vi "Configure Standard Waveform.vi"(0 "VISA resource name":refnum<visa-resource-name>, 1 "Waveform Function (0: Sine)":u16(ring) items=["Sine", "Square", "Ramp", "DC", "Pulse", "Arb"], 2 "Channel (1:Channel 1)":i32(ring)=1 items=["Channel 1"=1, "Channel 2"=2], 5 "Amplitude (1.0 Vpp)":dbl=1.0 format="%#.3f", 7 "Frequency (1000 Hz)":dbl=1000.0 format="%#.6g", 9 "DC Offset (0.00 V)":dbl, 11 "error in (no error)":errorcluster, 12 "Phase (0.0 degrees)":dbl=0.002 min=-360.0 max=360.0 format="%#.1g") -> (4 "VISA resource name out":refnum<visa-resource-name>, 15 "error out":errorcluster)   [LabVIEW 2015, in "SDG X Series.lvlib"]
doc: "Selects the waveform shape, frequency, amplitude, offset, and phase for standard waveforms (including Sine, Square, Ramp, Pulse, DC and Arb).\n\nNotes: \nTo configure other parameters for pulse waveforms please run the Configure Pulse VI. \nTo configure noise waveform please run the Configure Noise VI.\nTo configure other parameters for arbitrary waveforms please run the Create Arbitrary Waveform. \nTo configure PRBS waveform please run the Configure PRBS Waveform VI."
uses:
  <instrlib>/SDG X Series/SDG X Series.lvlib
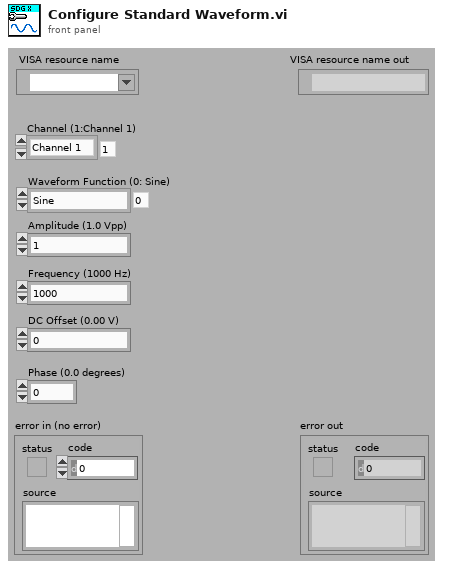
[diagram p1: front panel]
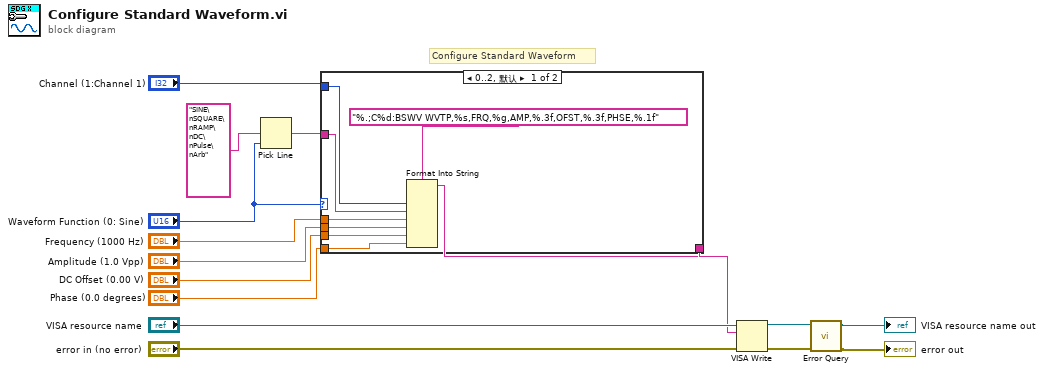
[diagram p0: block diagram]
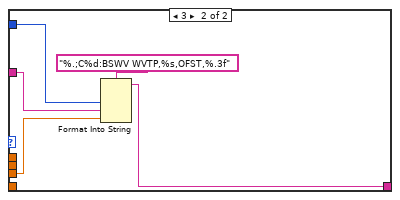
[diagram p2: hidden frame]
diagram:
  # "Configure Standard Waveform"
  n1 = Pick Line(multi-line string="SINE\nSQUARE\nRAMP\nDC\nPulse\nArb", line index="Waveform Function (0: Sine)") -> (output string=w14:string)  [unwired: 1 in]
  n2 = case shown="0..2, 默认" "Waveform Function (0: Sine)" {
    tunnel: w14 -> [w23 w26]
    tunnel: [w21 w24] -> w11
    tunnel: "Phase (0.0 degrees)" -> [w20 _]
    tunnel: "DC Offset (0.00 V)" -> [w19 w25]
    tunnel: "Amplitude (1.0 Vpp)" -> [w18 _]
    tunnel: "Frequency (1000 Hz)" -> [w17 _]
    tunnel: "Channel (1:Channel 1)" -> [w16 w27]
    frame 0..2, Default {
      n3 = Format Into String(format string="%.;C%d:BSWV WVTP,%s,FRQ,%g,AMP,%.3f,OFST,%.3f,PHSE,%.1f", w16, w23, w17, w18, w19, w20) -> (resulting string=w21:string)  [unwired: 2 in, 1 out]
    }
    frame 3 {
      n4 = Format Into String(format string="%.;C%d:BSWV WVTP,%s,OFST,%.3f", w27, w26, w25) -> (resulting string=w24:string)  [unwired: 2 in, 1 out]
    }
  }
  n5 = VISA Write(VISA resource name="VISA resource name", write buffer=w11, error in (no error)="error in (no error)") -> (VISA resource name out=w6:refnum<visa-resource-name>, error out=w5:errorcluster)  [unwired: 1 out]
  n6 = call <instrlib>:"Error Query.vi"("error in (no error)"=w5, "VISA resource name"=w6) -> ("error out"=→"error out":errorcluster, "VISA resource name out"=→"VISA resource name out":refnum<visa-resource-name>)  [unwired: 6 in, 2 out]
